vi "Prod - Session.vi"(8 "Error In":errorcluster, 11 "Prod-Data In":T3={"Queue_Producer"=refnum, "Queue_Consumer"=refnum, "To_GUI-Error_message"=refnum, "Rx-Data"=[], "Tx-Data"=[], "Console log"="", "Communication Settings"={"Tx Protocol"=enum."Not Active", "Rx Protocol"=enum."Serial", "Serial"={"Tx Port"="", "Rx Port"="", "Baud rate"=8, "Parity"=enum."Space", "Data bits"=0, "Stop bits"=0, "Flow control"=enum."None", "Tx Resource"="", "Rx Resource"=""}, "MIDI Device"={"Input uDevice ID"=0, "Output uDevice ID"=0, "hmidiout Handle"=0, "hmidiin Handle"=0}, "Bluetooth"={"Dummy"=""}, "USB"={"Dummy"=""}}, "MIDI-Messages"=[], "Queue_Session"=refnum, "To_GUI-Pre-Session"=refnum, "To_GUI-Producer"=refnum, "Tx Info"={"Datatype"=[], "Bytesize"=[], "Strings"=[], "ByteSum"=0}, "Payload"=variant, "Timout-Time[ms]"=0, "To_GUI-Session"=refnum, "CPU(ms)"=0}) -> (0 "Error Out":errorcluster, 3 "Prod-Data Out":T3={"Queue_Producer"=refnum, "Queue_Consumer"=refnum, "To_GUI-Error_message"=refnum, "Rx-Data"=[], "Tx-Data"=[], "Console log"="", "Communication Settings"={"Tx Protocol"=enum."Not Active", "Rx Protocol"=enum."Serial", "Serial"={"Tx Port"="", "Rx Port"="", "Baud rate"=8, "Parity"=enum."Space", "Data bits"=0, "Stop bits"=0, "Flow control"=enum."None", "Tx Resource"="", "Rx Resource"=""}, "MIDI Device"={"Input uDevice ID"=0, "Output uDevice ID"=0, "hmidiout Handle"=0, "hmidiin Handle"=0}, "Bluetooth"={"Dummy"=""}, "USB"={"Dummy"=""}}, "MIDI-Messages"=[], "Queue_Session"=refnum, "To_GUI-Pre-Session"=refnum, "To_GUI-Producer"=refnum, "Tx Info"={"Datatype"=[], "Bytesize"=[], "Strings"=[], "ByteSum"=0}, "Payload"=variant, "Timout-Time[ms]"=0, "To_GUI-Session"=refnum, "CPU(ms)"=0})   [LabVIEW 2019]
doc: "Description of VI"
uses:
  Controls/Producer-Data.ctl
  Common/Controls/Application_Message.ctl
  Common/Controls/Application_State.ctl
  Common/Controls/Communication_Settings.ctl
  Common/Controls/Communication_Protocols.ctl
  MIDI/Controls/MIDI-Message_Array.ctl
  MIDI/Controls/MIDI-Message_Cluster.ctl
  MIDI/Controls/Meta_Commands.ctl
  Controls/Prod - Tx_Info.ctl
  Controls/Session_State.ctl
  <vilib>/Utility/error.llb/DialogType.ctl
  Controls/Session_Data.ctl
  Consumer/Controls/Transfer_Data.ctl
  1da9ccfe-625d-42f9-b153-cb953530b974.vi
panel:
  in  "Control Tab":T1(tab)
  out "Process bar":i32(slide) scale=-1.0..2.0
  out "Tx-finished?":bool
  out "Session State:":T2
  out "Received":string
  out "Transmitted":string
  out "Console Out":string
  out "To Send":i32
  out "Sent":i32
  out "Error Message":string
  out "VI-filename":string
  out "VI Path":path
  out "Code Size":u32
  out "Revision Number":u32
  in  "Tool Bar:Visible":bool
  in  "Execution:Show Front Panel On Call":bool
  out "VI-Name":string
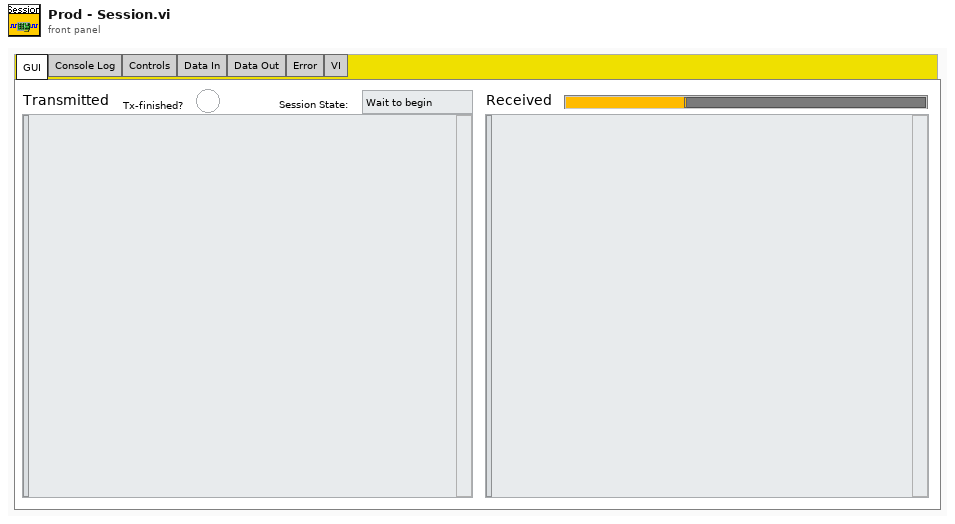
[diagram p1: front panel]
types:
  T1 = enum32{"GUI", "Console Log", "Controls", "Data In", "Data Out", "Error", "VI"}
  T2 = typedef "Session_State.ctl" = enum16{"Wait to begin", "Active Session", "Pause", "Wait for Response", "Stop", "Restart", "Inspect", "Exit"}
  T3 = typedef "Producer-Data.ctl" = cluster{"Queue_Producer":refnum<queue>, "Queue_Consumer":refnum<queue>, "To_GUI-Error_message":refnum<user-event>, "Rx-Data":i8[], "Tx-Data":i8[], "Console log":string, "Communication Settings":T4, "MIDI-Messages":T6, "Queue_Session":refnum<queue>, "To_GUI-Pre-Session":refnum<user-event>, "To_GUI-Producer":refnum<user-event>, "Tx Info":T9, "Payload":variant, "Timout-Time[ms]":i32, "To_GUI-Session":refnum<user-event>, "CPU(ms)":u32}
  T4 = typedef "Communication_Settings.ctl" = cluster{"Tx Protocol":T5, "Rx Protocol":T5, "Serial":cluster{"Tx Port":refnum<visa-resource-name>, "Rx Port":refnum<visa-resource-name>, "Baud rate":i32, "Parity":enum16{"None", "Odd", "Even", "Mark", "Space"}, "Data bits":i32, "Stop bits":i32, "Flow control":enum16{"None", "XON/XOFF", "RTS/CTS", "XON/XOFF & RTS/CTS", "DTR/DSR", "XON/XOFF & DTR/DSR"}, "Tx Resource":refnum<visa-resource-name>, "Rx Resource":refnum<visa-resource-name>}, "MIDI Device":cluster{"Input uDevice ID":u32, "Output uDevice ID":u32, "hmidiout Handle":i32, "hmidiin Handle":i32}, "Bluetooth":cluster{"Dummy":string}, "USB":cluster{"Dummy":string}}
  T5 = typedef "Communication_Protocols.ctl" = enum16{"Serial", "Bluetooth", "USB-MIDI", "MIDI (Audio Device)", "Not Active"}
  T6 = typedef "MIDI-Message_Array.ctl" = T7[]
  T7 = typedef "MIDI-Message_Cluster.ctl" = cluster{"Message Name":string, "Meta value":i32, "Datastring":string, "Datatype":T8}
  T8 = typedef "Meta_Commands.ctl" = enum16{"No Data", "Pause", "Loop", "Wait for Rx", "Delay", "Break", "MIDI"}
  T9 = typedef "Prod - Tx_Info.ctl" = cluster{"Datatype":T8[], "Bytesize":i32[], "Strings":string[], "ByteSum":i32}
  T10 = typedef "Session_Data.ctl" = cluster{"MIDI-Messages":T6, "Rx-Data":i8[], "Tx-Data":i8[], "Session States":T2, "Tx Index":i32, "Communication Settings":T4, "Timout-Time[ms]":i32, "Payload":variant, "Queue_Session":refnum<queue>, "To_GUI-Session":refnum<user-event>, "No More\nData":bool, "Queue_Consumer":refnum<queue>, "MIDI-Messages Log":T6, "Console log":string}
  T11 = typedef "DialogType.ctl" = u16
  T12 = typedef "Application_State.ctl" = enum16{"Idle", "Initiate", "MH Load Messages", "Prepare for Tx", "Settings", "Com Session", "Receive", "Data", "Uninitialize", "Quit Message", "Export Send"}
  T13 = typedef "Application_Message.ctl" = cluster{"Application State":T12, "Payload":variant}
  T14 = typedef "Transfer_Data.ctl" = cluster{"Tx-Data":i8[], "Rx-Data":i8[], "MIDI-Message log":T6}
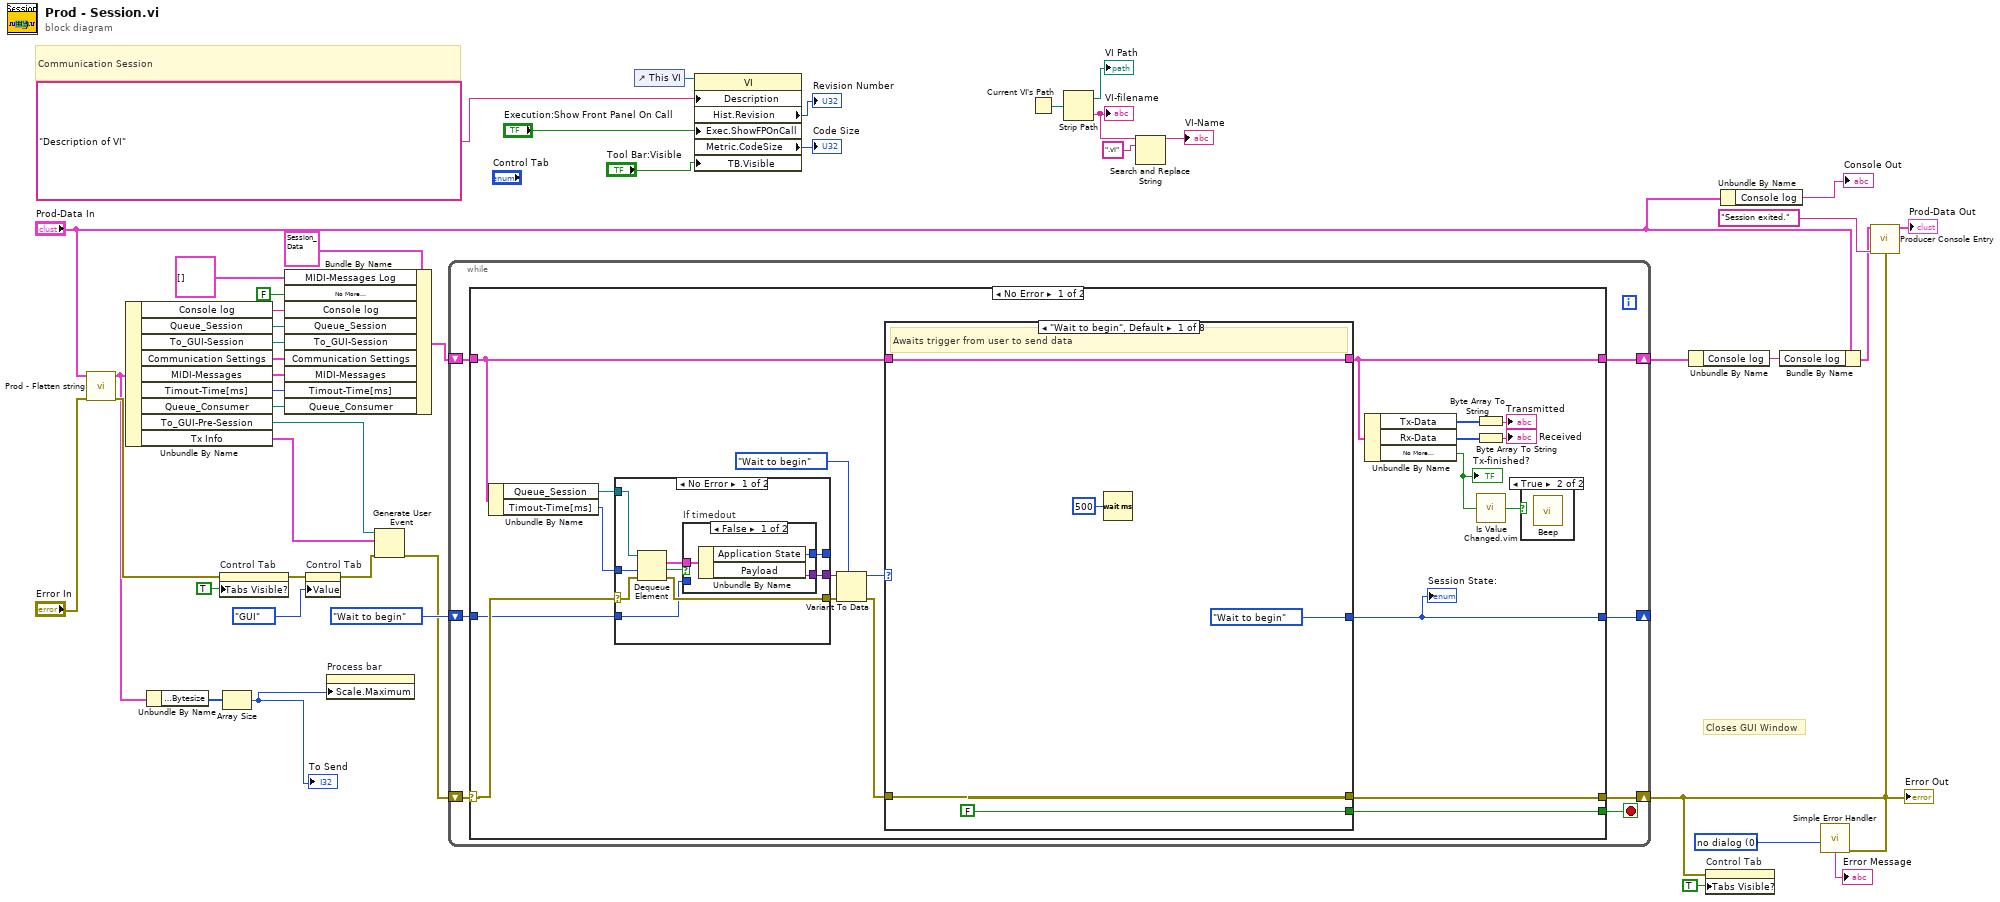
[diagram p0: block diagram]
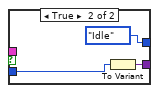
[diagram p3: hidden frame]
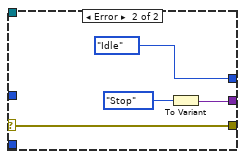
[diagram p4: hidden frame]
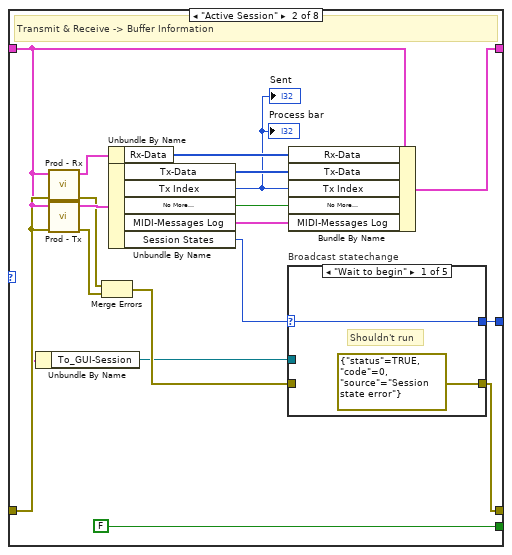
[diagram p5: hidden frame]
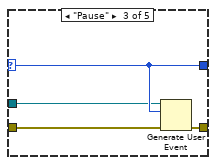
[diagram p7: hidden frame]
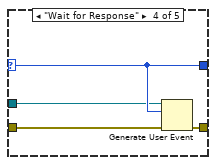
[diagram p8: hidden frame]
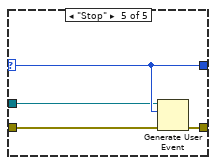
[diagram p9: hidden frame]
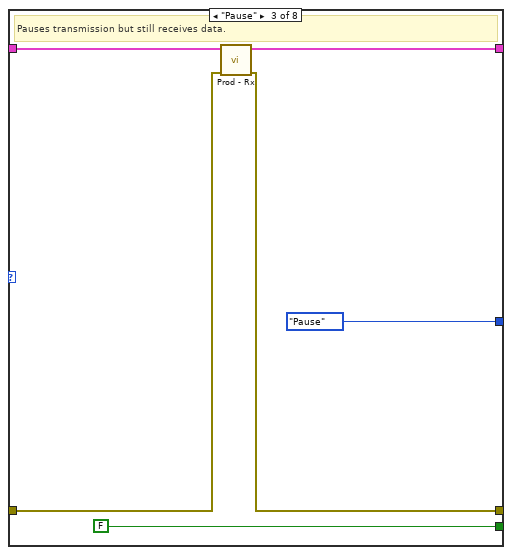
[diagram p10: hidden frame]
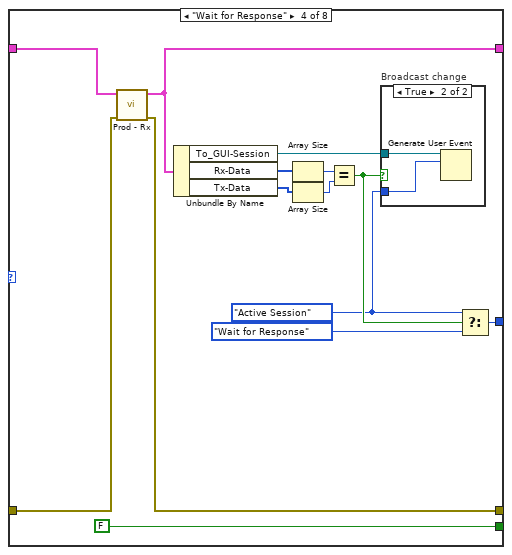
[diagram p11: hidden frame]
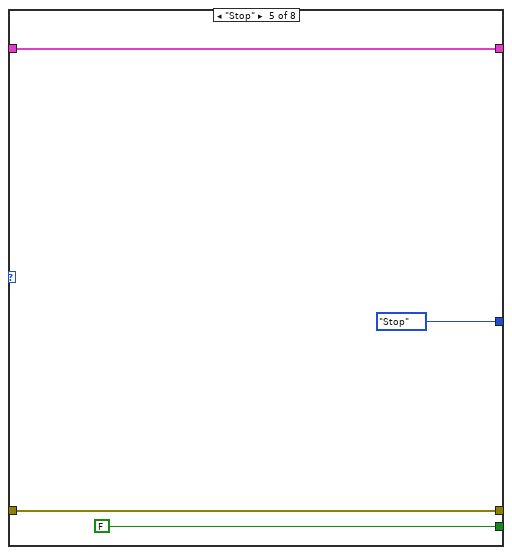
[diagram p13: hidden frame]
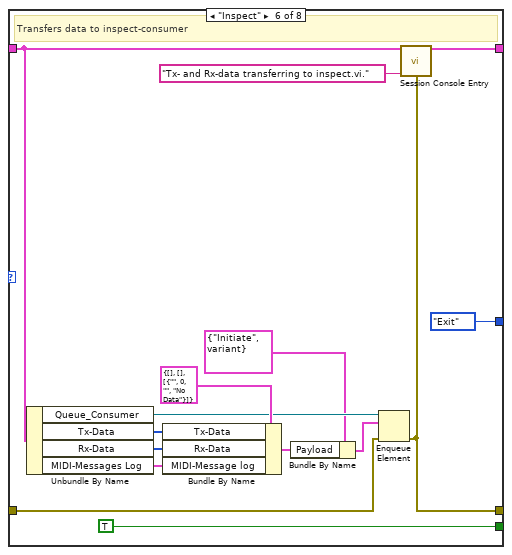
[diagram p14: hidden frame]
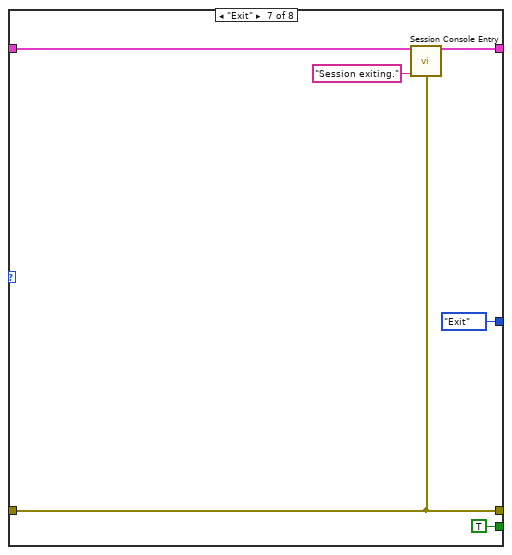
[diagram p15: hidden frame]
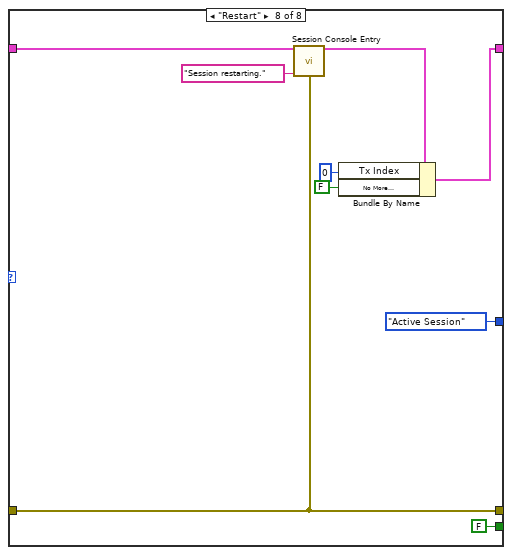
[diagram p16: hidden frame]
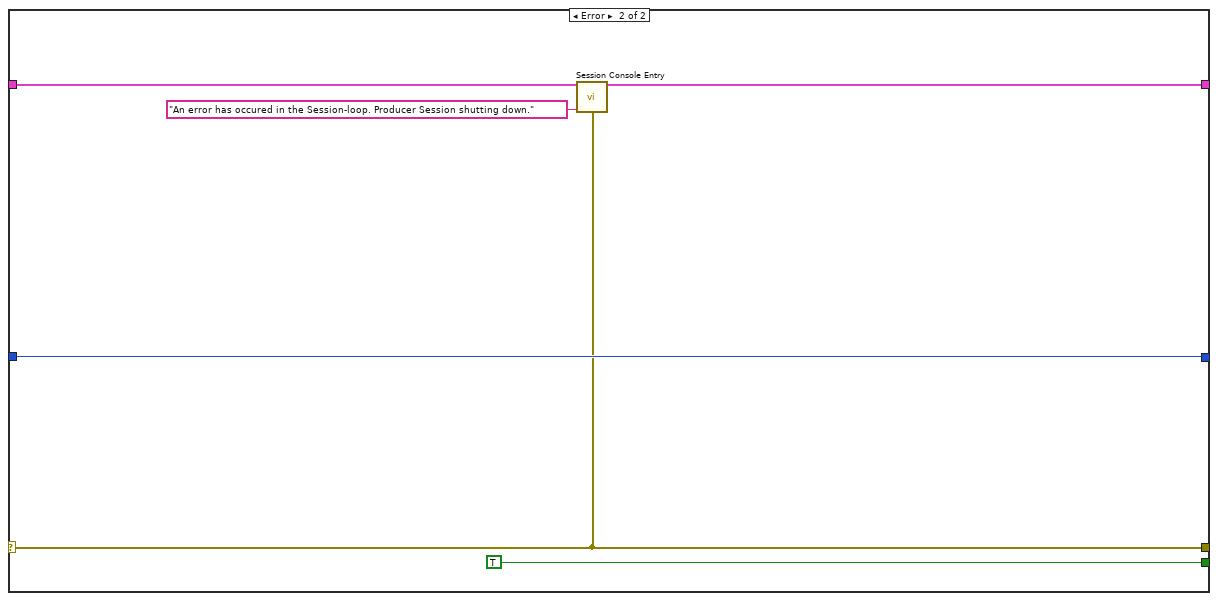
[diagram p17: hidden frame]
diagram:
  w32 = T11 0 items=["no dialog", "OK message", "continue or stop message", "OK message + warnings", "continue/stop + warnings"] ("type of dialog (OK msg:1)")
  # "Closes GUI Window"
  # "Communication Session"
  n1 = call "Prod - Flatten string.vi"("Error In"="Error In", "Prod-Data In"="Prod-Data In") -> ("Error Out"=w14:errorcluster, "Prod-Data Out"=w3:T3)  [unwired: 8 in]
  n2 = Unbundle By Name(w3) -> ("Console log"=w8:string, "Queue_Session"=w29:refnum<queue>, "To_GUI-Session"=w26:refnum<user-event>, "Communication Settings"=w24:T4, "MIDI-Messages"=w25:T6, "Timout-Time[ms]"=w19:i32, "Queue_Consumer"=w11:refnum<queue>, "To_GUI-Pre-Session"=w12:refnum<user-event>, "Tx Info"=w21:T9)
  n3 = Unbundle By Name(w3) -> ("Tx Info.Bytesize"=w2:i32[])
  n4 = property on="Control Tab" class="TabCtl (strict)"(error in=w14, "Tabs Visible?"=TRUE) -> (error out=w16:errorcluster)  [unwired: 1 in, 1 out]
  n5 = Array Size(array=w2) -> (size(s)=w1:i32)
  "To Send" <- w1
  n6 = Bundle By Name(cluster=T10 {"MIDI-Messages"=[], "Rx-Data"=[], "Tx-Data"=[], "Session States"=enum."Wait to begin", "Tx Index"=0, "Communication Settings"={"Tx Protocol"=enum."Not Active", "Rx Protocol"=enum."Serial", "Serial"={"Tx Port"="", "Rx Port"="", "Baud rate"=8, "Parity"=enum."Space", "Data bits"=0, "Stop bits"=0, "Flow control"=enum."None", "Tx Resource"="", "Rx Resource"=""}, "MIDI Device"={"Input uDevice ID"=0, "Output uDevice ID"=0, "hmidiout Handle"=0, "hmidiin Handle"=0}, "Bluetooth"={"Dummy"=""}, "USB"={"Dummy"=""}}, "Timout-Time[ms]"=0, "Payload"=variant, "Queue_Session"=refnum, "To_GUI-Session"=refnum, "No More\nData"=FALSE, "Queue_Consumer"=refnum, "MIDI-Messages Log"=[], "Console log"=""} ("Session Data"), "MIDI-Messages Log"=T6 [], "No More\nData"=FALSE ("No More\nData"), "Console log"=w8, "Queue_Session"=w29, "To_GUI-Session"=w26, "Communication Settings"=w24, "MIDI-Messages"=w25, "Timout-Time[ms]"=w19, "Queue_Consumer"=w11) -> (w23:T10)
  n7 = property on="Control Tab" class="TabCtl (strict)"(error in=w16, "Value"=T1."GUI" ("Control Tab")) -> (error out=w15:errorcluster)  [unwired: 1 in, 1 out]
  n8 = property on="Process bar" class="Slide (strict)"("Scale.Maximum"=w1) -> ()  [unwired: 2 in, 2 out]
  n9 = Generate User Event(user event=w12, event data cluster=w21, error in=w15) -> (error out=w20:errorcluster)  [unwired: 1 in, 1 out]
  n10 = while {
    shift-right: [w50] -> _
    shift-left: Session_State."Wait to begin" ("Enum") -> [w51]
    shift-right: [w48] -> w7
    shift-left: w23 -> [w49]
    shift-right: [w52] -> w13
    shift-left: w20 -> [w53]
    stop <- w47 stop-if-true
    n11 = case shown="No Error" w53 {
      selector: w53 -> [w69 w188]
      tunnel: [w73 w188] -> w52
      tunnel: w51 -> [w63 w193]
      tunnel: [w57 w193] -> w50
      tunnel: w49 -> [w71 w191]
      tunnel: [w62 w190] -> w48
      tunnel: [w72 TRUE] -> w47
      frame No Error {
        n12 = Unbundle By Name(w71) -> ("Queue_Session"=w70:refnum<queue>, "Timout-Time[ms]"=w68:i32)
        n13 = case shown="No Error" w69 {
          selector: w69 -> [w79 w92]
          tunnel: [w78 w92] -> w66
          tunnel: [w81 Application_State."Idle" ("Data_Type")] -> _
          tunnel: [w80 w89] -> w67
          tunnel: w70 -> [w77 _]
          tunnel: w68 -> [w76 _]
          tunnel: w63 -> [w74 _]
          frame No Error {
            n14 = Dequeue Element(queue=w77, timeout in ms (-1)=w76, error in (no error)=w79) -> (element=w82:T13, timed out?=w75:bool, error out=w78:errorcluster)  [unwired: 1 out]
            n15 = case "If timedout" shown="False" w75 {
              tunnel: w82 -> [w85 _]
              tunnel: [w84 Application_State."Idle" ("Data_Type")] -> w81
              tunnel: [w83 w87] -> w80
              tunnel: w74 -> [_ w86]
              frame False {
                n16 = Unbundle By Name(w85) -> ("Application State"=w84:T12, "Payload"=w83:variant)
              }
              frame True {
                n17 = To Variant(anything=w86) -> (Variant=w87:variant)
              }
            }
          }
          frame Error {
            n18 = To Variant(anything=Session_State."Stop" ("Enum")) -> (Variant=w89:variant)
          }
        }
        n19 = Variant To Data(error in=w66, type=Session_State."Wait to begin" ("Enum"), Variant=w67) -> (data=w64:T2, error out=w56:errorcluster)
        n20 = case shown="\"Wait to begin\", Default" w64 {
          tunnel: [Session_State."Wait to begin" ("Enum") w107 Session_State."Pause" ("Enum") w150 Session_State."Stop" ("Enum") Session_State."Exit" ("Enum") Session_State."Exit" ("Enum") Session_State."Active Session" ("Enum")] -> w57
          tunnel: w71 -> [w94 w104 w137 w149 w156 w161 w176 w183]
          tunnel: [w94 w112 w136 w146 w156 w160 w175 w187] -> w62
          tunnel: w56 -> [w95 w110 w135 w148 w155 w162 w173 w180]
          tunnel: [w95 w105 w134 w147 w155 w158 w173 w180] -> w73
          tunnel: [FALSE FALSE FALSE FALSE FALSE TRUE TRUE FALSE] -> w72
          frame "Wait to begin", Default {
            # "Awaits trigger from user to send data"
            n21 = Wait (ms)(milliseconds to wait=u32 500) -> ()  [unwired: 1 out]
          }
          frame "Active Session" {
            # "Transmit & Receive -> Buffer Information"
            n22 = Unbundle By Name(w104) -> ("To_GUI-Session"=w103:refnum<user-event>)
            n23 = call "Prod - Rx.vi"("Error In"=w110, "Session Data In"=w104) -> ("Error Out"=w109:errorcluster, "Session Data Out"=w114:T10)  [unwired: 8 in]
            n24 = call "Prod - Tx.vi"("Error In"=w110, "Session Data In"=w104) -> ("Error Out"=w108:errorcluster, "Session Data Out"=w115:T10)  [unwired: 8 in]
            n25 = Merge Errors(w109, w108) -> (w106:errorcluster)
            n26 = Unbundle By Name(w114) -> ("Rx-Data"=w99:i8[])
            n27 = Unbundle By Name(w115) -> ("Tx-Data"=w113:i8[], "Tx Index"=w98:i32, "No More\nData"=w102:bool, "MIDI-Messages Log"=w100:T6, "Session States"=w101:T2)
            "Process bar" <- w98
            "Sent" <- w98
            n28 = case "Broadcast statechange" shown="\"Wait to begin\"" w101 {
              selector: w101 -> [w117 w119 w123 w127 w131]
              tunnel: [w117 w119 w123 w127 w131] -> w107
              tunnel: w106 -> [_ w118 w122 w126 w130]
              tunnel: [errorcluster {"status"=TRUE, "code"=0, "source"="Session state error"} ("error out") w118 w121 w125 w129] -> w105
              tunnel: w103 -> [_ _ w120 w124 w128]
              frame "Wait to begin" {
                # "Shouldn't run"
              }
              frame "Active Session", Default {
              }
              frame "Pause" {
                n29 = Generate User Event(user event=w120, event data cluster=w123, error in=w122) -> (error out=w121:errorcluster)  [unwired: 1 in, 1 out]
              }
              frame "Wait for Response" {
                n30 = Generate User Event(user event=w124, event data cluster=w127, error in=w126) -> (error out=w125:errorcluster)  [unwired: 1 in, 1 out]
              }
              frame "Stop" {
                n31 = Generate User Event(user event=w128, event data cluster=w131, error in=w130) -> (error out=w129:errorcluster)  [unwired: 1 in, 1 out]
              }
            }
            n32 = Bundle By Name(cluster=w104, "Rx-Data"=w99, "Tx-Data"=w113, "Tx Index"=w98, "No More\nData"=w102, "MIDI-Messages Log"=w100) -> (w112:T10)
          }
          frame "Pause" {
            # "Pauses transmission but still receives data."
            n33 = call "Prod - Rx.vi"("Error In"=w135, "Session Data In"=w137) -> ("Error Out"=w134:errorcluster, "Session Data Out"=w136:T10)  [unwired: 8 in]
          }
          frame "Wait for Response" {
            w138 = Session_State."Active Session" ("t")
            n34 = call "Prod - Rx.vi"("Error In"=w148, "Session Data In"=w149) -> ("Error Out"=w147:errorcluster, "Session Data Out"=w146:T10)  [unwired: 8 in]
            n35 = Unbundle By Name(w146) -> ("To_GUI-Session"=w139:refnum<user-event>, "Rx-Data"=w145:i8[], "Tx-Data"=w144:i8[])
            n36 = Array Size(array=w145) -> (size(s)=w143:i32)
            n37 = Array Size(array=w144) -> (size(s)=w142:i32)
            n38 = Equal?(x=w143, y=w142) -> (x = y?=w140:bool)
            n39 = case "Broadcast change" shown="True" w140 {
              tunnel: w139 -> [_ w153]
              tunnel: w138 -> [_ w152]
              frame False {
              }
              frame True {
                n40 = Generate User Event(user event=w153, event data cluster=w152) -> ()  [unwired: 2 in, 2 out]
              }
            }
            n41 = Select(t=w138, s=w140, f=Session_State."Wait for Response" ("Enum")) -> (s? t:f=w150:T2)
          }
          frame "Stop" {
          }
          frame "Inspect" {
            # "Transfers data to inspect-consumer"
            n42 = Unbundle By Name(w161) -> ("Queue_Consumer"=w166:refnum<queue>, "Tx-Data"=w169:i8[], "Rx-Data"=w168:i8[], "MIDI-Messages Log"=w167:T6)
            n43 = Bundle By Name(cluster=T14 {"Tx-Data"=[], "Rx-Data"=[], "MIDI-Message log"=[{"Message Name"="", "Meta value"=0, "Datastring"="", "Datatype"=enum."No Data"}]}, "Tx-Data"=w169, "Rx-Data"=w168, "MIDI-Message log"=w167) -> (w164:T14)
            n44 = Bundle By Name(cluster=T13 {"Application State"=enum."Initiate", "Payload"=variant} ("element"), "Payload"=w164) -> (w163:T13)
            n45 = Enqueue Element(queue=w166, element=w163, error in (no error)=w162) -> (error out=w158:errorcluster)  [unwired: 1 in, 2 out]
            n46 = call "Session Console Entry.vi"("Session Data In"=w161, "Console Entry"="Tx- and Rx-data transferring to inspect.vi.", "Error In"=w158) -> ("Session Data 2"=w160:T10)  [unwired: 12 in]
          }
          frame "Exit" {
            n47 = call "Session Console Entry.vi"("Session Data In"=w176, "Console Entry"="Session exiting.", "Error In"=w173) -> ("Session Data 2"=w175:T10)  [unwired: 12 in]
          }
          frame "Restart" {
            n48 = call "Session Console Entry.vi"("Session Data In"=w183, "Console Entry"="Session restarting.", "Error In"=w180) -> ("Session Data 2"=w182:T10)  [unwired: 12 in]
            n49 = Bundle By Name(cluster=w182, "Tx Index"=0, "No More\nData"=FALSE ("No More\nData")) -> (w187:T10)
          }
        }
        "Session State:" <- w57
        n50 = Unbundle By Name(w62) -> ("Tx-Data"=w61:i8[], "Rx-Data"=w60:i8[], "No More\nData"=w54:bool)
        "Tx-finished?" <- w54
        n51 = Byte Array To String(unsigned byte array=w61) -> (string=→"Transmitted":string)
        n52 = Byte Array To String(unsigned byte array=w60) -> (string=→"Received":string)
        n53 = call "Is Value Changed.vim"("value"=w54) -> ("changed or first call?"=w55:bool)
        n54 = case shown="True" w55 {
          frame False {
          }
          frame True {
            n55 = call <vilib>:"Beep.vi"() -> ()  [unwired: 12 in]
          }
        }
      }
      frame Error {
        n56 = call "Session Console Entry.vi"("Session Data In"=w191, "Console Entry"="An error has occured in the Session-loop. Producer Session shutting down.", "Error In"=w188) -> ("Session Data 2"=w190:T10)  [unwired: 12 in]
      }
    }
  }
  "Error Out" <- w13
  n57 = control-ref of="This VI"() -> (w39:refnum<vi>)
  n58 = property class="VI"(reference=w39, "Description"="Description of VI", "Exec.ShowFPOnCall"="Execution:Show Front Panel On Call", "TB.Visible"="Tool Bar:Visible") -> ("Hist.Revision"=→"Revision Number":u32, "Metric.CodeSize"=→"Code Size":u32)  [unwired: 1 in, 2 out]
  n59 = Current VI's Path() -> (path=w46:path)
  n60 = Strip Path(path=w46) -> (stripped path=→"VI Path":path, name=w36:string)
  "VI-filename" <- w36
  n61 = Search and Replace String(input string=w36, search string=".vi") -> (result string=→"VI-Name":string)  [unwired: 6 in, 3 out]
  n62 = Unbundle By Name(w7) -> ("Console log"=w6:string)
  n63 = property on="Control Tab" class="TabCtl (strict)"(error in=w13, "Tabs Visible?"=TRUE) -> ()  [unwired: 1 in, 2 out]
  n64 = Unbundle By Name("Prod-Data In") -> ("Console log"=→"Console Out":string)
  n65 = Bundle By Name(cluster="Prod-Data In", "Console log"=w6) -> (w4:T3)
  n66 = call <vilib>:"Simple Error Handler.vi"("type of dialog (OK msg:1)"=w32, "error in (no error)"=w13) -> ("message"=→"Error Message":string)  [unwired: 3 in, 4 out]
  n67 = call "Producer Console Entry.vi"("Prod-Data In"=w4, "Console Entry"="Session exited.", "Error In"=w13) -> ("Prod-Data Out"=→"Prod-Data Out":T3)  [unwired: 12 in]
